vi "Rotate.vi"(7 "Direction of Rotation":T1, 8 "error in (no error)":errorcluster, 10 "Rotation Angle (Deg.)":dbl, 11 "Angle in":refnum<class "Angle.lvclass">) -> (0 "error out":errorcluster, 2 "New Angle":dbl, 3 "Angle out":refnum<class "Angle.lvclass">)   [LabVIEW 2011, in "Angle.lvclass"]
doc: "Calculates a new angle that is the old angle rotated by the rotation angle."
uses:
  Angle.lvclass
  TypeDefs/DirectionOfRotation.ctl
  Angle.lvclass/Angle.ctl
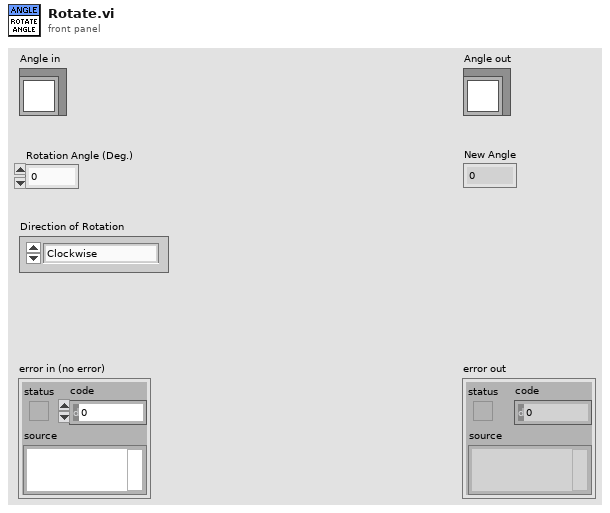
[diagram p1: front panel]
types:
  T1 = typedef "DirectionOfRotation.ctl" = enum16{"Clockwise", "Counter-Clockwise"}
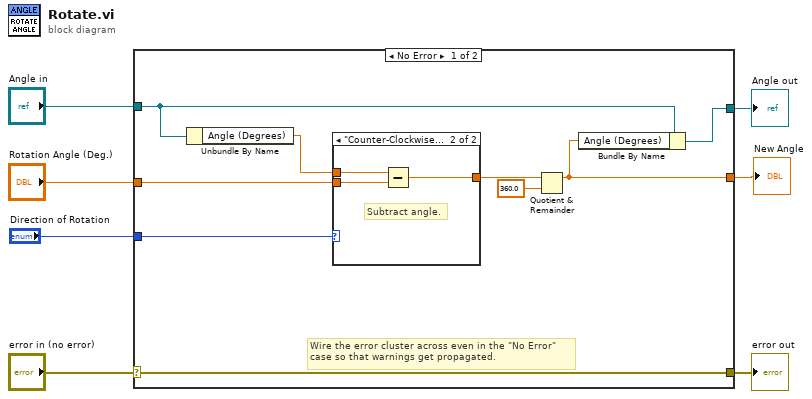
[diagram p0: block diagram]
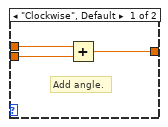
[diagram p2: hidden frame]
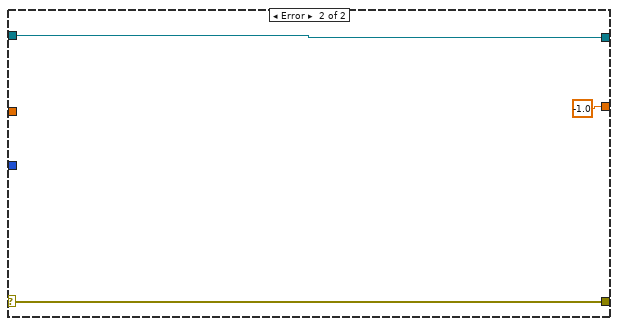
[diagram p3: hidden frame]
diagram:
  n1 = case shown="No Error" "error in (no error)" {
    selector: "error in (no error)" -> [w16 w25]
    tunnel: [w16 w25] -> w6
    tunnel: [w13 w24] -> w4
    tunnel: "Angle in" -> [w14 w24]
    tunnel: "Rotation Angle (Deg.)" -> [w8 _]
    tunnel: [w12 -1.0] -> w2
    tunnel: "Direction of Rotation" -> [w11 _]
    frame No Error {
      # "Wire the error cluster across even in the \"No Error\"\ncase so that warnings get propagated."
      n2 = Unbundle By Name(w14) -> ("Angle (Degrees)"=w9:dbl)
      n3 = case shown="\"Counter-Clockwise\"" w11 {
        tunnel: [w19 w22] -> w10
        tunnel: w9 -> [w18 w21]
        tunnel: w8 -> [w17 w20]
        frame "Clockwise", Default {
          # "Add angle."
          n4 = Add(x=w18, y=w17) -> (x+y=w19:dbl)
        }
        frame "Counter-Clockwise" {
          # "Subtract angle."
          n5 = Subtract(x=w21, y=w20) -> (x-y=w22:dbl)
        }
      }
      n6 = Quotient & Remainder(x=w10, y=360.0) -> (x-y*floor(x/y)=w12:dbl)  [unwired: 1 out]
      n7 = Bundle By Name(cluster=w14, "Angle (Degrees)"=w12) -> (w13:refnum<class "Angle.lvclass">)
    }
    frame Error {
    }
  }
  "error out" <- w6
  "Angle out" <- w4
  "New Angle" <- w2
